vi "Lookup Group.vi"(8 "error in (no error)":errorcluster, 10 "Group Name":string, 11 "ChannelService in":refnum<class "ChannelService.lvclass">) -> (0 "error out":errorcluster, 2 "Group":refnum<class "Group.lvclass">, 3 "ChannelService out":refnum<class "ChannelService.lvclass">)   [LabVIEW 2020, in "Vecto.lvlib" / "ChannelService.lvclass"]
uses:
  ChannelService.lvclass
  Group/Group.lvclass
  GroupValue/GroupValue.lvclass
  C:/Program Files (x86)/National Instruments/LabVIEW 2024/vi.lib/IlluminatedG/IG Promises/Promises/Value/Value.lvclass
  Lookup Group Data.ctl
  <vilib>/IlluminatedG/IG Promises/Promises/Promise/Promise.lvclass
  ChannelService.lvclass/ChannelService.ctl
  <vilib>/IlluminatedG/IG Promises/Promises/Promise/Promise.lvclass/Promise.ctl
  <vilib>/IlluminatedG/IG Promises/Promises/Future/Future.lvclass/Future.ctl
  GroupValue/GroupValue.lvclass/GroupValue.ctl
  <vilib>/IlluminatedG/IG Promises/Promises/Future/Future.lvclass
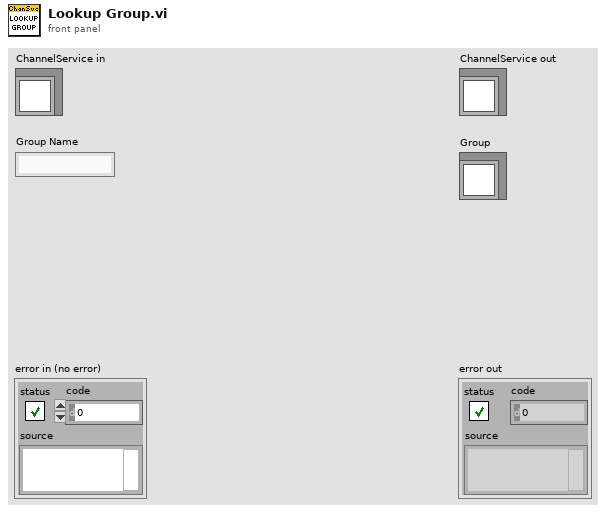
[diagram p1: front panel]
types:
  T1 = typedef "Vecto.lvlib/ChannelService.lvclass/Lookup Group Data.ctl" = cluster{"Group Name":string, "Promise":refnum<class "Promise.lvclass">}
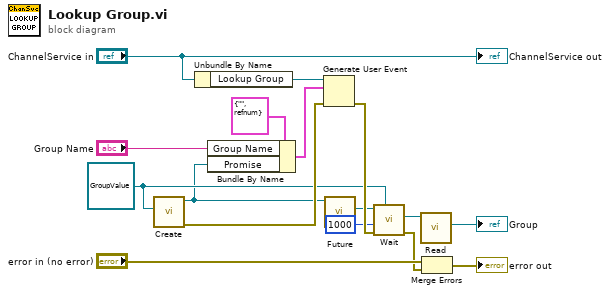
[diagram p0: block diagram]
diagram:
  w12 = refnum<class "GroupValue.lvclass"> refnum ("Vecto.lvlib:GroupValue.lvclass")
  n1 = call <vilib>:"Create.vi"("Result Type"=w12) -> ("error out"=w15:errorcluster, "Promise"=w5:refnum<class "Promise.lvclass">)  [unwired: 9 in]
  n2 = Unbundle By Name("ChannelService in") -> ("Lookup Group"=w8:refnum<user-event>)
  n3 = Bundle By Name(cluster=T1 {"Group Name"="", "Promise"=refnum} ("event data"), "Group Name"="Group Name", "Promise"=w5) -> (w4:T1)
  n4 = Generate User Event(user event=w8, event data cluster=w4, error in=w15) -> (error out=w16:errorcluster)  [unwired: 1 in, 1 out]
  n5 = call <vilib>:"Future.vi"("Promise in"=w5) -> ("Future"=w13:refnum<class "Future.lvclass">)  [unwired: 9 in, 1 out]
  n6 = call <vilib>:"Wait.vi"("Result Type"=w12, "error in (no error)"=w16, "Timeout mS (-1)"=1000, "Future in"=w13) -> ("error out"=w1:errorcluster, "Result"=w10:refnum<class "GroupValue.lvclass">)  [unwired: 6 in]
  n7 = call "Read.vi"("GroupValue in"=w10) -> ("Group"=→"Group":refnum<class "Group.lvclass">)  [unwired: 10 in]
  n8 = Merge Errors("error in (no error)", w1) -> (→"error out":errorcluster)
  "ChannelService out" <- "ChannelService in"
